vi "subHistogram_ApplyScaleLimit.vi"(8 "Error in":errorcluster, 10 "IntGraph Refnum":refnum<vi>, 11 "XYGraph Refnum":refnum<vi>) -> (0 "Error out":errorcluster, 3 "Scale":cluster{"Scale.Min":i32, "Scale.Max":i32}={"Scale.Min"=100, "Scale.Max"=100} {"Scale.Max" min=1 max=5000 step=1; "Scale.Min" min=1 max=5000 step=1})   [LabVIEW 2015]
panel:
  # "Apply scale limit and get scale cursor"
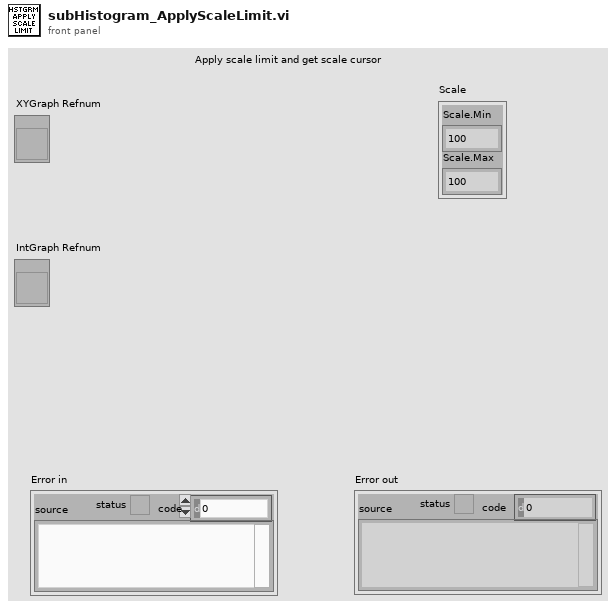
[diagram p1: front panel]
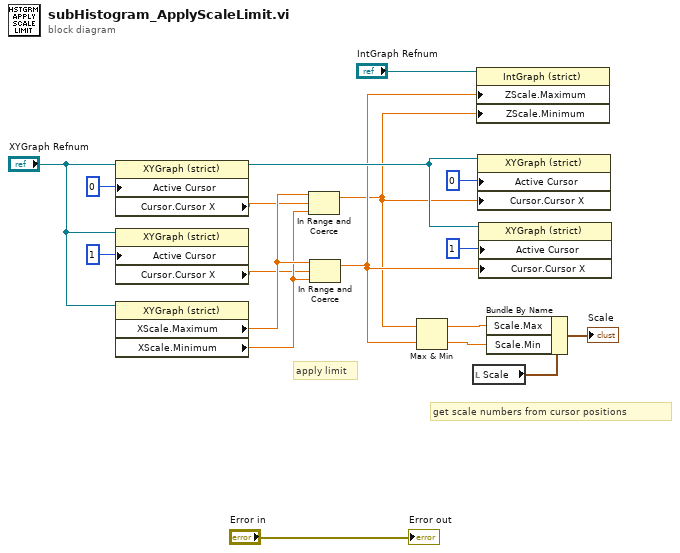
[diagram p0: block diagram]
diagram:
  # "get scale numbers from cursor positions"
  # "apply limit"
  n1 = property on="Property Node" class="XYGraph (strict)"(reference="XYGraph Refnum", "Active Cursor"=u32 0) -> (reference out=w14:refnum<vi>, "Cursor.Cursor X"=w6:dbl)  [unwired: 1 in, 1 out]
  n2 = property on="Property Node" class="XYGraph (strict)"(reference="XYGraph Refnum", "Active Cursor"=u32 1) -> ("Cursor.Cursor X"=w5:dbl)  [unwired: 1 in, 2 out]
  n3 = property on="Property Node" class="XYGraph (strict)"(reference="XYGraph Refnum") -> ("XScale.Maximum"=w8:dbl, "XScale.Minimum"=w7:dbl)  [unwired: 1 in, 2 out]
  n4 = In Range and Coerce(upper limit=w8, x=w6, lower limit=w7) -> (coerced(x)=w1:dbl)  [unwired: 1 out]
  n5 = In Range and Coerce(upper limit=w8, x=w5, lower limit=w7) -> (coerced(x)=w2:dbl)  [unwired: 1 out]
  n6 = Max & Min(x=w1, y=w2) -> (max(x,y)=w12:dbl, min(x,y)=w11:dbl)
  n7 = local read "Scale"() -> (w13:cluster{"Scale.Min":i32, "Scale.Max":i32})
  n8 = property on="Property Node" class="IntGraph (strict)"(reference="IntGraph Refnum", "ZScale.Maximum"=w2, "ZScale.Minimum"=w1) -> ()  [unwired: 1 in, 2 out]
  n9 = property on="Property Node" class="XYGraph (strict)"(reference=w14, "Active Cursor"=u32 0, "Cursor.Cursor X"=w1) -> ()  [unwired: 1 in, 2 out]
  n10 = property on="Property Node" class="XYGraph (strict)"(reference=w14, "Active Cursor"=u32 1, "Cursor.Cursor X"=w2) -> ()  [unwired: 1 in, 2 out]
  n11 = Bundle By Name(cluster=w13, "Scale.Max"=w12, "Scale.Min"=w11) -> (→"Scale":cluster{"Scale.Min":i32, "Scale.Max":i32})
  "Error out" <- "Error in"
